vi "Results Checker.vi"(7 "Test Name":T3, 9 "Model Name":T5, 10 "Results":T6, 11 "Results Cluster":T4) -> (3 "Results Cluster out":T4)   [LabVIEW 2017]
uses:
  controls/AC Results.ctl
  controls/Model Name.ctl
  controls/Results Cluster.ctl
  controls/Result Checker.ctl
  controls/All Specs.ctl
  controls/Specifications.ctl
  GV/Specs.vi
panel:
  in  "All Specs":T1={"LH"={"Go Up"={"Min Speed"=10.0, "Max Speed"=250.0, "Min Time"=0.5, "Max Time"=4.3, "Min Run Current"=0.0, "Max Run Current"=10.0, "Min Stall Current"=0.0, "Max Stall Current"=25.0, "Min Stall Force"=170.0, "Max Stall Force"=320.0, "Min Stroke"=254.4, "Max Stroke"=270.4}, "Go Down"={"Min Speed"=10.0, "Max Speed"=250.0, "Min Travel Time"=0.5, "Max Travel Time"=4.3, "Min Run Current"=0.0, "Max Run Current"=10.0}, "Shipping"={"Min Distance"=5.0, "Max Distance"=15.0, "Setpoint"=5.0}, "Anti-Pinch"={"Min Force"=5.0, "Max Force"=15.0}}, "RH"={"Go Up"={"Min Speed"=10.0, "Max Speed"=250.0, "Min Time"=0.5, "Max Time"=4.3, "Min Run Current"=0.0, "Max Run Current"=10.0, "Min Stall Current"=0.0, "Max Stall Current"=25.0, "Min Stall Force"=170.0, "Max Stall Force"=320.0, "Min Stroke"=254.4, "Max Stroke"=270.4}, "Go Down"={"Min Speed"=10.0, "Max Speed"=250.0, "Min Travel Time"=0.5, "Max Travel Time"=4.3, "Min Run Current"=0.0, "Max Run Current"=10.0}, "Shipping"={"Min Distance"=5.0, "Max Distance"=15.0, "Setpoint"=5.0}, "Anti-Pinch"={"Min Force"=5.0, "Max Force"=15.0}}, "W 601 FR RH Std"={"Go Up"={"Min Speed"=10.0, "Max Speed"=250.0, "Min Time"=0.5, "Max Time"=4.3, "Min Run Current"=0.0, "Max Run Current"=10.0, "Min Stall Current"=0.0, "Max Stall Current"=25.0, "Min Stall Force"=170.0, "Max Stall Force"=320.0, "Min Stroke"=254.4, "Max Stroke"=270.4}, "Go Down"={"Min Speed"=10.0, "Max Speed"=250.0, "Min Travel Time"=0.5, "Max Travel Time"=4.3, "Min Run Current"=0.0, "Max Run Current"=10.0}, "Shipping"={"Min Distance"=5.0, "Max Distance"=15.0, "Setpoint"=5.0}, "Anti-Pinch"={"Min Force"=5.0, "Max Force"=15.0}}, "W 601 FR LH Std"={"Go Up"={"Min Speed"=10.0, "Max Speed"=250.0, "Min Time"=0.5, "Max Time"=4.3, "Min Run Current"=0.0, "Max Run Current"=10.0, "Min Stall Current"=0.0, "Max Stall Current"=25.0, "Min Stall Force"=170.0, "Max Stall Force"=320.0, "Min Stroke"=254.4, "Max Stroke"=270.4}, "Go Down"={"Min Speed"=10.0, "Max Speed"=250.0, "Min Travel Time"=0.5, "Max Travel Time"=4.3, "Min Run Current"=0.0, "Max Run Current"=10.0}, "Shipping"={"Min Distance"=5.0, "Max Distance"=15.0, "Setpoint"=5.0}, "Anti-Pinch"={"Min Force"=5.0, "Max Force"=15.0}}, "W 601 RR RH Std"={"Go Up"={"Min Speed"=10.0, "Max Speed"=250.0, "Min Time"=0.5, "Max Time"=4.3, "Min Run Current"=0.0, "Max Run Current"=10.0, "Min Stall Current"=0.0, "Max Stall Current"=25.0, "Min Stall Force"=170.0, "Max Stall Force"=320.0, "Min Stroke"=254.4, "Max Stroke"=270.4}, "Go Down"={"Min Speed"=10.0, "Max Speed"=250.0, "Min Travel Time"=0.5, "Max Travel Time"=4.3, "Min Run Current"=0.0, "Max Run Current"=10.0}, "Shipping"={"Min Distance"=5.0, "Max Distance"=15.0, "Setpoint"=5.0}, "Anti-Pinch"={"Min Force"=5.0, "Max Force"=15.0}}, "W 601 RR LH Std"={"Go Up"={"Min Speed"=10.0, "Max Speed"=250.0, "Min Time"=0.5, "Max Time"=4.3, "Min Run Current"=0.0, "Max Run Current"=10.0, "Min Stall Current"=0.0, "Max Stall Current"=25.0, "Min Stall Force"=170.0, "Max Stall Force"=320.0, "Min Stroke"=254.4, "Max Stroke"=270.4}, "Go Down"={"Min Speed"=10.0, "Max Speed"=250.0, "Min Travel Time"=0.5, "Max Travel Time"=4.3, "Min Run Current"=0.0, "Max Run Current"=10.0}, "Shipping"={"Min Distance"=5.0, "Max Distance"=15.0, "Setpoint"=5.0}, "Anti-Pinch"={"Min Force"=5.0, "Max Force"=15.0}}, "W 601 FR RH AP"={"Go Up"={"Min Speed"=10.0, "Max Speed"=250.0, "Min Time"=0.5, "Max Time"=4.3, "Min Run Current"=0.0, "Max Run Current"=10.0, "Min Stall Current"=0.0, "Max Stall Current"=25.0, "Min Stall Force"=170.0, "Max Stall Force"=320.0, "Min Stroke"=254.4, "Max Stroke"=270.4}, "Go Down"={"Min Speed"=10.0, "Max Speed"=250.0, "Min Travel Time"=0.5, "Max Travel Time"=4.3, "Min Run Current"=0.0, "Max Run Current"=10.0}, "Shipping"={"Min Distance"=5.0, "Max Distance"=15.0, "Setpoint"=5.0}, "Anti-Pinch"={"Min Force"=5.0, "Max Force"=15.0}}, "W 601 FR LH AP"={"Go Up"={"Min Speed"=10.0, "Max Speed"=250.0, "Min Time"=0.5, "Max Time"=4.3, "Min Run Current"=0.0, "Max Run Current"=10.0, "Min Stall Current"=0.0, "Max Stall Current"=25.0, "Min Stall Force"=170.0, "Max Stall Force"=320.0, "Min Stroke"=254.4, "Max Stroke"=270.4}, "Go Down"={"Min Speed"=10.0, "Max Speed"=250.0, "Min Travel Time"=0.5, "Max Travel Time"=4.3, "Min Run Current"=0.0, "Max Run Current"=10.0}, "Shipping"={"Min Distance"=5.0, "Max Distance"=15.0, "Setpoint"=5.0}, "Anti-Pinch"={"Min Force"=5.0, "Max Force"=15.0}}, "W 601 RR RH AP"={"Go Up"={"Min Speed"=10.0, "Max Speed"=250.0, "Min Time"=0.5, "Max Time"=4.3, "Min Run Current"=0.0, "Max Run Current"=10.0, "Min Stall Current"=0.0, "Max Stall Current"=25.0, "Min Stall Force"=170.0, "Max Stall Force"=320.0, "Min Stroke"=254.4, "Max Stroke"=270.4}, "Go Down"={"Min Speed"=10.0, "Max Speed"=250.0, "Min Travel Time"=0.5, "Max Travel Time"=4.3, "Min Run Current"=0.0, "Max Run Current"=10.0}, "Shipping"={"Min Distance"=5.0, "Max Distance"=15.0, "Setpoint"=5.0}, "Anti-Pinch"={"Min Force"=5.0, "Max Force"=15.0}}, "W 601 RR LH AP"={"Go Up"={"Min Speed"=10.0, "Max Speed"=250.0, "Min Time"=0.5, "Max Time"=4.3, "Min Run Current"=0.0, "Max Run Current"=10.0, "Min Stall Current"=0.0, "Max Stall Current"=25.0, "Min Stall Force"=170.0, "Max Stall Force"=320.0, "Min Stroke"=254.4, "Max Stroke"=270.4}, "Go Down"={"Min Speed"=10.0, "Max Speed"=250.0, "Min Travel Time"=0.5, "Max Travel Time"=4.3, "Min Run Current"=0.0, "Max Run Current"=10.0}, "Shipping"={"Min Distance"=5.0, "Max Distance"=15.0, "Setpoint"=5.0}, "Anti-Pinch"={"Min Force"=5.0, "Max Force"=15.0}}}
  # "SPECIFICATIONS"
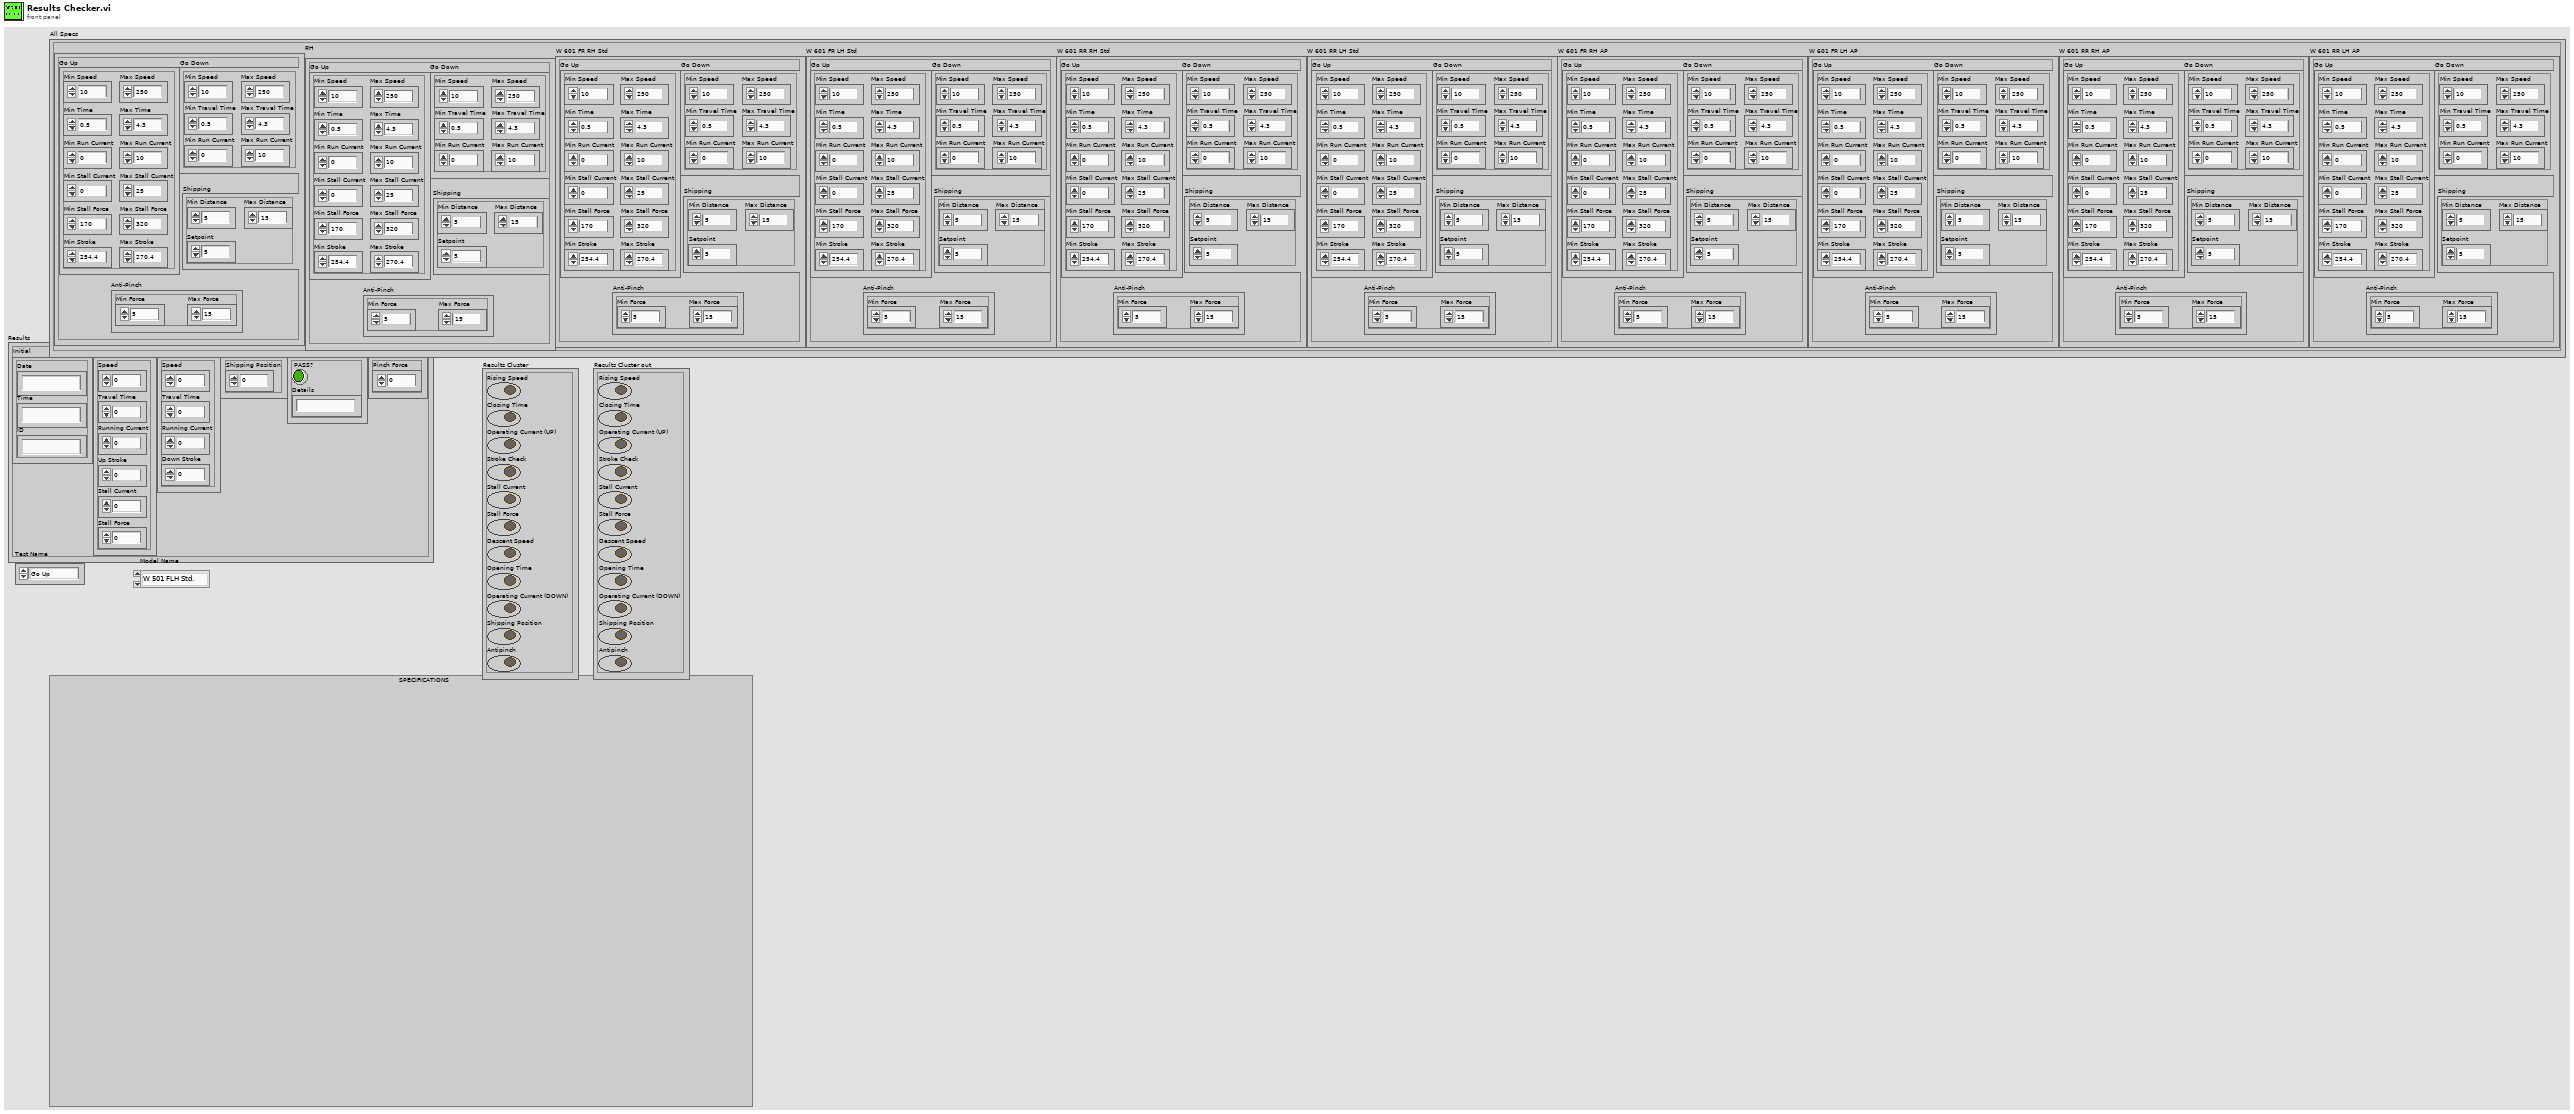
[diagram p1: front panel]
types:
  T1 = typedef "All Specs.ctl" = cluster{"LH":T2, "RH":T2, "W 601 FR RH Std":T2, "W 601 FR LH Std":T2, "W 601 RR RH Std":T2, "W 601 RR LH Std":T2, "W 601 FR RH AP":T2, "W 601 FR LH AP":T2, "W 601 RR RH AP":T2, "W 601 RR LH AP":T2}
  T2 = typedef "Specifications.ctl" = cluster{"Go Up":cluster{"Min Speed":dbl, "Max Speed":dbl, "Min Time":dbl, "Max Time":dbl, "Min Run Current":dbl, "Max Run Current":dbl, "Min Stall Current":dbl, "Max Stall Current":dbl, "Min Stall Force":dbl, "Max Stall Force":dbl, "Min Stroke":dbl, "Max Stroke":dbl}, "Go Down":cluster{"Min Speed":dbl, "Max Speed":dbl, "Min Travel Time":dbl, "Max Travel Time":dbl, "Min Run Current":dbl, "Max Run Current":dbl}, "Shipping":cluster{"Min Distance":dbl, "Max Distance":dbl, "Setpoint":dbl}, "Anti-Pinch":cluster{"Min Force":dbl, "Max Force":dbl}}
  T3 = typedef "Result Checker.ctl" = enum16{"Go Up", "Go Down", "Stall Force", "Shipping Position", "Antipinch"}
  T4 = typedef "Results Cluster.ctl" = cluster{"Rising Speed":bool, "Closing Time":bool, "Operating Current (UP)":bool, "Stroke Check":bool, "Stall Current":bool, "Stall Force":bool, "Descent Speed":bool, "Opening Time":bool, "Operating Current (DOWN)":bool, "Shipping Position":bool, "Antipinch":bool}
  T5 = typedef "Model Name.ctl" = enum16{"W 501 FLH Std.", "W 501 FRH Std.", "W 601 FR RH Std", "W 601 FR LH Std", "W 601 RR RH Std", "W 601 RR LH Std", "W 601 FR RH AP", "W 601 FR LH AP", "W 601 RR RH AP", "W 601 RR LH AP"}
  T6 = typedef "AC Results.ctl" = cluster{"Initial":cluster{"Date":string, "Time":string, "ID":string}, "Go Up":cluster{"Speed":dbl, "Travel Time":dbl, "Running Current":dbl, "Up Stroke":dbl, "Stall Current":dbl, "Stall Force":dbl}, "Go Down":cluster{"Speed":dbl, "Travel Time":dbl, "Running Current":dbl, "Down Stroke":dbl}, "Shipping Position":cluster{"Shipping Position":dbl}, "Results":cluster{"PASS?":bool, "Details":string}, "Antipinch":cluster{"Pinch Force":dbl}}
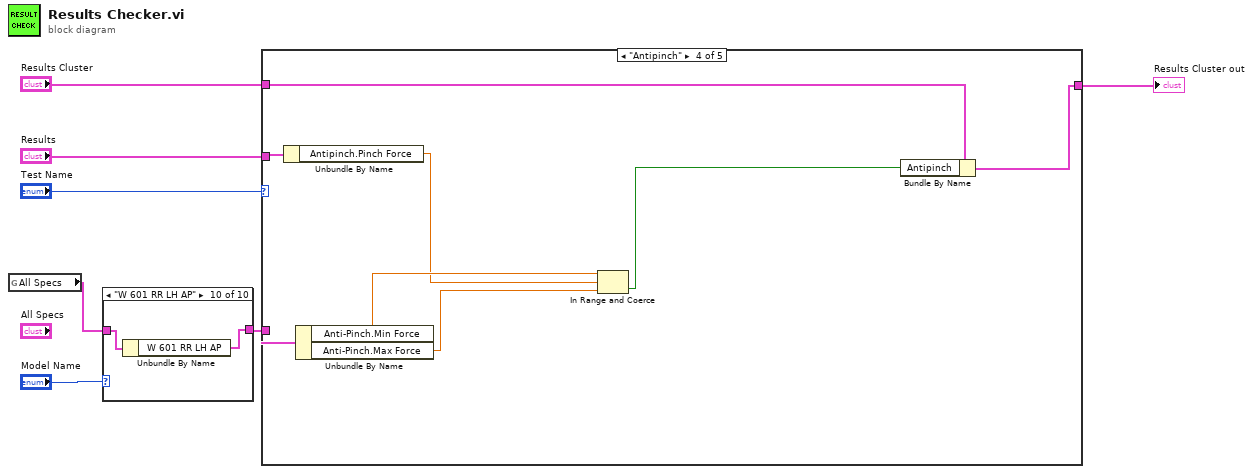
[diagram p0: block diagram]
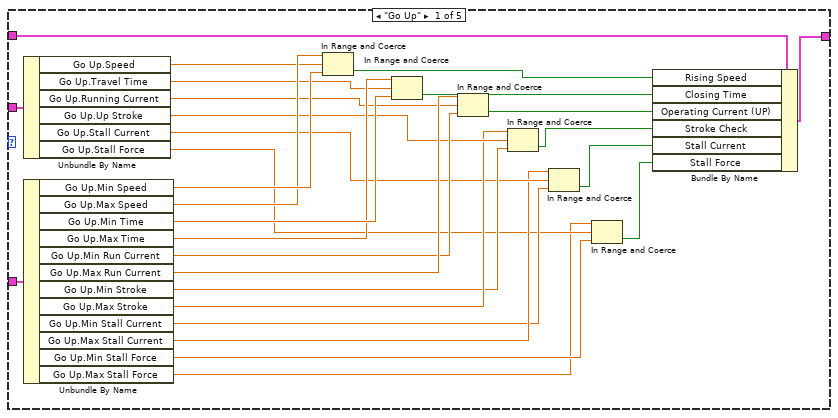
[diagram p2: hidden frame]
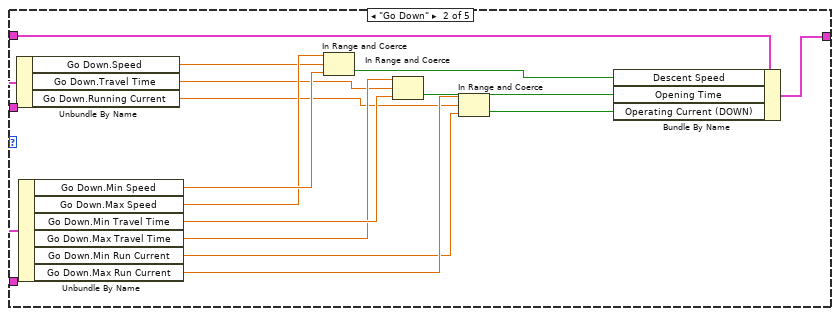
[diagram p3: hidden frame]
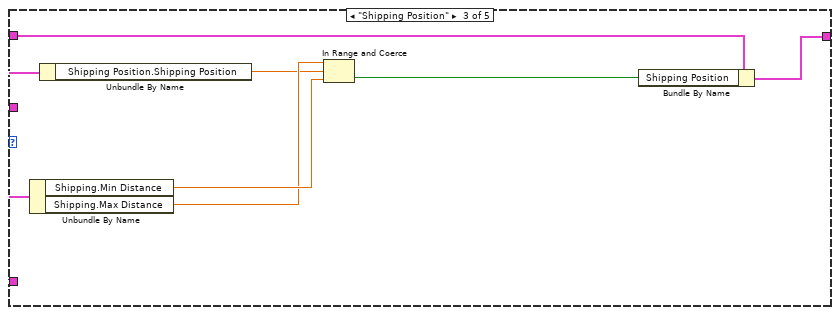
[diagram p4: hidden frame]
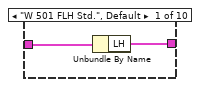
[diagram p6: hidden frame]
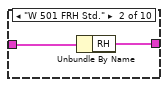
[diagram p7: hidden frame]
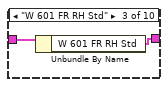
[diagram p8: hidden frame]
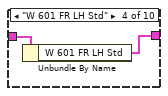
[diagram p9: hidden frame]
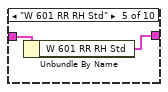
[diagram p10: hidden frame]
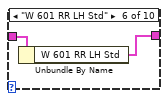
[diagram p11: hidden frame]
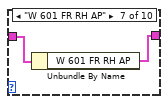
[diagram p12: hidden frame]
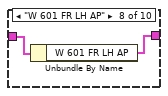
[diagram p13: hidden frame]
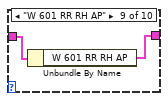
[diagram p14: hidden frame]
diagram:
  n1 = global read "Specs.vi" "All Specs"() -> (w1:T1)
  n2 = case shown="\"W 601 RR LH AP\"" "Model Name" {
    tunnel: w1 -> [w9 w11 w13 w15 w17 w19 w21 w23 w25 w27]
    tunnel: [w8 w10 w12 w14 w16 w18 w20 w22 w24 w26] -> w3
    frame "W 501 FLH Std.", Default {
      n3 = Unbundle By Name(w9) -> ("LH"=w8:T2)
    }
    frame "W 501 FRH Std." {
      n4 = Unbundle By Name(w11) -> ("RH"=w10:T2)
    }
    frame "W 601 FR RH Std" {
      n5 = Unbundle By Name(w13) -> ("W 601 FR RH Std"=w12:T2)
    }
    frame "W 601 FR LH Std" {
      n6 = Unbundle By Name(w15) -> ("W 601 FR LH Std"=w14:T2)
    }
    frame "W 601 RR RH Std" {
      n7 = Unbundle By Name(w17) -> ("W 601 RR RH Std"=w16:T2)
    }
    frame "W 601 RR LH Std" {
      n8 = Unbundle By Name(w19) -> ("W 601 RR LH Std"=w18:T2)
    }
    frame "W 601 FR RH AP" {
      n9 = Unbundle By Name(w21) -> ("W 601 FR RH AP"=w20:T2)
    }
    frame "W 601 FR LH AP" {
      n10 = Unbundle By Name(w23) -> ("W 601 FR LH AP"=w22:T2)
    }
    frame "W 601 RR RH AP" {
      n11 = Unbundle By Name(w25) -> ("W 601 RR RH AP"=w24:T2)
    }
    frame "W 601 RR LH AP" {
      n12 = Unbundle By Name(w27) -> ("W 601 RR LH AP"=w26:T2)
    }
  }
  n13 = case shown="\"Antipinch\"" "Test Name" {
    tunnel: "Results" -> [w55 w71 w79 w86 _]
    tunnel: w3 -> [w54 w70 w78 w87 _]
    tunnel: "Results Cluster" -> [w53 w69 w77 w82 w88]
    tunnel: [w52 w68 w76 w80 w88] -> w4
    frame "Go Up" {
      n14 = Unbundle By Name(w55) -> ("Go Up.Speed"=w49:dbl, "Go Up.Travel Time"=w44:dbl, "Go Up.Running Current"=w41:dbl, "Go Up.Up Stroke"=w39:dbl, "Go Up.Stall Current"=w34:dbl, "Go Up.Stall Force"=w31:dbl)
      n15 = Unbundle By Name(w54) -> ("Go Up.Min Speed"=w51:dbl, "Go Up.Max Speed"=w50:dbl, "Go Up.Min Time"=w46:dbl, "Go Up.Max Time"=w45:dbl, "Go Up.Min Run Current"=w42:dbl, "Go Up.Max Run Current"=w43:dbl, "Go Up.Min Stroke"=w37:dbl, "Go Up.Max Stroke"=w38:dbl, "Go Up.Min Stall Current"=w32:dbl, "Go Up.Max Stall Current"=w33:dbl, "Go Up.Min Stall Force"=w29:dbl, "Go Up.Max Stall Force"=w28:dbl)
      n16 = In Range and Coerce(upper limit=w50, x=w49, lower limit=w51) -> (In Range?=w48:bool)  [unwired: 1 out]
      n17 = In Range and Coerce(upper limit=w45, x=w44, lower limit=w46) -> (In Range?=w47:bool)  [unwired: 1 out]
      n18 = In Range and Coerce(upper limit=w43, x=w41, lower limit=w42) -> (In Range?=w40:bool)  [unwired: 1 out]
      n19 = In Range and Coerce(upper limit=w38, x=w39, lower limit=w37) -> (In Range?=w36:bool)  [unwired: 1 out]
      n20 = In Range and Coerce(upper limit=w33, x=w34, lower limit=w32) -> (In Range?=w35:bool)  [unwired: 1 out]
      n21 = In Range and Coerce(upper limit=w28, x=w31, lower limit=w29) -> (In Range?=w30:bool)  [unwired: 1 out]
      n22 = Bundle By Name(cluster=w53, "Rising Speed"=w48, "Closing Time"=w47, "Operating Current (UP)"=w40, "Stroke Check"=w36, "Stall Current"=w35, "Stall Force"=w30) -> (w52:T4)
    }
    frame "Go Down" {
      n23 = Unbundle By Name(w71) -> ("Go Down.Speed"=w65:dbl, "Go Down.Travel Time"=w60:dbl, "Go Down.Running Current"=w57:dbl)
      n24 = Unbundle By Name(w70) -> ("Go Down.Min Speed"=w67:dbl, "Go Down.Max Speed"=w66:dbl, "Go Down.Min Travel Time"=w62:dbl, "Go Down.Max Travel Time"=w61:dbl, "Go Down.Min Run Current"=w58:dbl, "Go Down.Max Run Current"=w59:dbl)
      n25 = In Range and Coerce(upper limit=w66, x=w65, lower limit=w67) -> (In Range?=w64:bool)  [unwired: 1 out]
      n26 = In Range and Coerce(upper limit=w61, x=w60, lower limit=w62) -> (In Range?=w63:bool)  [unwired: 1 out]
      n27 = In Range and Coerce(upper limit=w59, x=w57, lower limit=w58) -> (In Range?=w56:bool)  [unwired: 1 out]
      n28 = Bundle By Name(cluster=w69, "Descent Speed"=w64, "Opening Time"=w63, "Operating Current (DOWN)"=w56) -> (w68:T4)
    }
    frame "Shipping Position" {
      n29 = Unbundle By Name(w78) -> ("Shipping.Min Distance"=w75:dbl, "Shipping.Max Distance"=w74:dbl)
      n30 = Unbundle By Name(w79) -> ("Shipping Position.Shipping Position"=w73:dbl)
      n31 = In Range and Coerce(upper limit=w74, x=w73, lower limit=w75) -> (In Range?=w72:bool)  [unwired: 1 out]
      n32 = Bundle By Name(cluster=w77, "Shipping Position"=w72) -> (w76:T4)
    }
    frame "Antipinch" {
      n33 = Unbundle By Name(w86) -> ("Antipinch.Pinch Force"=w83:dbl)
      n34 = Unbundle By Name(w87) -> ("Anti-Pinch.Min Force"=w85:dbl, "Anti-Pinch.Max Force"=w84:dbl)
      n35 = In Range and Coerce(upper limit=w85, x=w83, lower limit=w84) -> (In Range?=w81:bool)  [unwired: 1 out]
      n36 = Bundle By Name(cluster=w82, "Antipinch"=w81) -> (w80:T4)
    }
    frame Default {
    }
  }
  "Results Cluster out" <- w4
